vi "LJStreamM read and log.vi"(0 "# Channels":i32=100 min=1, 1 "Scan Rate (Hz)":dbl=500.0 format="%.3f", 2 "# Scans On Graph":i32=1000 min=0, 3 "Update Channel Ref":bool, 4 "LJStreamM Front Panel References":T2, 5 "(LJM) Error In":errorcluster, 6 "Row Modification Options":T1={" Row #"=1, "Delete Row"=FALSE, "Insert Row"=FALSE} {"Row #" min=0 max=95}, 8 "Handle In":i32=43, 10 "start stream":bool caption="Start Stream") -> (9 "Handle Out":i32=43, 14 "Raw Value":dbl[](array[numeric])=[-0.0013667265884578228, 0.9637618064880371, -0.6710270047187805, -1.0797535181045532, -2.244410514831543, -2.9202396869659424, -3.8373279571533203, -4.381304740905762, -5.186929702758789, -5.547481536865234, -6.286360263824463, -6.849207401275635, -8.288508415222168, -9.301578521728516, 1.8125708103179932, -0.0013901632046326995, -0.0013901632046326995, -0.0014061988331377506, -0.001392630278132856, -0.0014173004310578108, -0.0013457569293677807, -0.0013704270822927356, -0.0013149193255230784, -0.0013260208070278168, -1.6386336088180542, -1.2051987648010254, -0.7538595199584961, -0.2919749915599823, 0.20884576439857483, 0.6676713228225708, 1.1433043479919434, 1.6328012943267822, -0.7485023736953735, -0.28742581605911255, 0.18301406502723694, 0.6747994422912598, 1.1796000003814697, 1.6914348602294922, 2.204704523086548, 2.7171919345855713, 0.29239073395729065, 0.7711177468299866, 1.2827318906784058, 1.7454545497894287, 2.2245850563049316, 2.724728584289551, 3.220463991165161, 3.7060885429382324, 1.3471759557724, 1.8994848728179932, 2.4582371711730957, 3.017115592956543, 3.568817377090454, 4.132509231567383, 4.696534633636475, 5.25940465927124, 2.4371588230133057, 2.9621644020080566, 3.493621826171875, 4.033999919891357, 4.572134494781494, 5.092087745666504, 5.614201545715332, 6.141404151916504, 3.54797101020813, 4.116397857666016, 4.69553279876709, 5.2544169425964355, 5.819548606872559, 6.3801727294921875, 6.980928897857666, 7.524782180786133, 4.545636177062988, 5.073090553283691, 5.603622913360596, 6.125936508178711, 6.640289306640625, 7.1512274742126465, 7.6685028076171875, 8.177851676940918, 5.359930992126465, 5.915652275085449, 6.470480442047119, 7.029056549072266, 7.650485038757324, 8.190069198608398, 8.722926139831543, 9.247248649597168, 6.308043956756592, 6.83182430267334, 7.344102382659912, 7.853759765625, 8.360687255859375, 8.86483383178711, 9.365800857543945, 9.856183052062988, 6.392543792724609, 6.943355083465576, 7.586986064910889, 8.126357078552246] format="%.6f", 15 "Scaled Value":dbl[](array[numeric])=[-0.0013667265884578228, 0.9637618064880371, -0.6710270047187805, -1.0797535181045532, -2.244410514831543, -2.9202396869659424, -3.8373279571533203, -4.381304740905762, -5.186929702758789, -5.547481536865234, -6.286360263824463, -6.849207401275635, -8.288508415222168, -9.301578521728516, 1.8125708103179932, -0.0013901632046326995, -0.0013901632046326995, -0.0014061988331377506, -0.001392630278132856, -0.0014173004310578108, -0.0013457569293677807, -0.0013704270822927356, -0.0013149193255230784, -0.0013260208070278168, -1.6386336088180542, -1.2051987648010254, -0.7538595199584961, -0.2919749915599823, 0.20884576439857483, 0.6676713228225708, 1.1433043479919434, 1.6328012943267822, -0.7485023736953735, -0.28742581605911255, 0.18301406502723694, 0.6747994422912598, 1.1796000003814697, 1.6914348602294922, 2.204704523086548, 2.7171919345855713, 0.29239073395729065, 0.7711177468299866, 1.2827318906784058, 1.7454545497894287, 2.2245850563049316, 2.724728584289551, 3.220463991165161, 3.7060885429382324, 1.3471759557724, 1.8994848728179932, 2.4582371711730957, 3.017115592956543, 3.568817377090454, 4.132509231567383, 4.696534633636475, 5.25940465927124, 2.4371588230133057, 2.9621644020080566, 3.493621826171875, 4.033999919891357, 4.572134494781494, 5.092087745666504, 5.614201545715332, 6.141404151916504, 3.54797101020813, 4.116397857666016, 4.69553279876709, 5.2544169425964355, 5.819548606872559, 6.3801727294921875, 6.980928897857666, 7.524782180786133, 4.545636177062988, 5.073090553283691, 5.603622913360596, 6.125936508178711, 6.640289306640625, 7.1512274742126465, 7.6685028076171875, 8.177851676940918, 5.359930992126465, 5.915652275085449, 6.470480442047119, 7.029056549072266, 7.650485038757324, 8.190069198608398, 8.722926139831543, 9.247248649597168, 6.308043956756592, 6.83182430267334, 7.344102382659912, 7.853759765625, 8.360687255859375, 8.86483383178711, 9.365800857543945, 9.856183052062988, 6.392543792724609, 6.943355083465576, 7.586986064910889, 8.126357078552246] format="%.6f", 16 "Last Error Message":string="No Error", 17 "Last Error Message Status":bool, 18 "Channel Setup Reference Out":refnum<vi>, 19 "(LJM) Error Out":errorcluster)   [LabVIEW 2026]
uses:
  Common Logger Controls/Channel Setup.ctl
  LJStreamM Front Panel References.ctl
  Common Logger Controls/Row Modification Options.ctl
  Common Logger VIs/LJM logger Globals.vi
panel:
  in  "Channel Setup":T3={"Name"=["AIN0", "AIN1", "AIN2", "AIN3", "AIN4", "AIN5", "AIN6", "AIN7", "AIN8", "AIN9", "AIN10", "AIN11", "AIN12", "AIN13", "AIN14", "AIN15", "AIN16", "AIN17", "AIN18", "AIN19", "AIN20", "AIN21", "AIN22", "AIN23", "AIN24", "AIN25", "AIN26", "AIN27", "AIN28", "AIN29", "AIN30", "AIN31", "AIN32", "AIN33", "AIN34", "AIN35", "AIN36", "AIN37", "AIN38", "AIN39", "AIN40", "AIN41", "AIN42", "AIN43", "AIN44", "AIN45", "AIN46", "AIN47", "AIN48", "AIN49", "AIN50", "AIN51", "AIN52", "AIN53", "AIN54", "AIN55", "AIN56", "AIN57", "AIN58", "AIN59", "AIN60", "AIN61", "AIN62", "AIN63", "AIN64", "AIN65", "AIN66", "AIN67", "AIN68", "AIN69", "AIN70", "AIN71", "AIN72", "AIN73", "AIN74", "AIN75", "AIN76", "AIN77", "AIN78", "AIN79", "AIN80", "AIN81", "AIN82", "AIN83", "AIN84", "AIN85", "AIN86", "AIN87", "AIN88", "AIN89", "AIN90", "AIN91", "AIN92", "AIN93", "AIN94", "AIN95", "AIN96", "AIN97", "AIN98", "AIN99"], "", "Scaling Equation"=["y=a", "y=b", "y=c", "y=d", "y=e", "y=f", "y=g", "y=h", "y=i", "y=j", "y=k", "y=l", "y=m", "y=n", "y=o", "y=p", "y=q", "y=r", "y=s", "y=t", "y=u", "y=v", "y=w", "y=x", "y=y", "y=z", "y=a2", "y=b2", "y=c2", "y=d2", "y=e2", "y=f2", "y=g2", "y=h2", "y=i2", "y=j2", "y=k2", "y=l2", "y=m2", "y=n2", "y=o2", "y=p2", "y=q2", "y=r2", "y=s2", "y=t2", "y=u2", "y=v2", "y=w2", "y=x2", "y=y2", "y=z2", "y=a3", "y=b3", "y=c3", "y=d3", "y=e3", "y=f3", "y=g3", "y=h3", "y=i3", "y=j3", "y=k3", "y=l3", "y=m3", "y=n3", "y=o3", "y=p3", "y=q3", "y=r3", "y=s3", "y=t3", "y=u3", "y=v3", "y=w3", "y=x3", "y=y3", "y=z3", "y=a4", "y=b4", "y=c4", "y=d4", "y=e4", "y=f4", "y=g4", "y=h4", "y=i4", "y=j4", "y=k4", "y=l4", "y=m4", "y=n4", "y=o4", "y=p4", "y=q4", "y=r4", "y=s4", "y=t4", "y=u4", "y=v4"], "", "Graph?"=[TRUE, TRUE, TRUE, TRUE, FALSE, FALSE, FALSE, FALSE, FALSE, FALSE, FALSE, FALSE, FALSE, FALSE, FALSE, FALSE, FALSE, FALSE, FALSE, FALSE, FALSE, FALSE, FALSE, FALSE, FALSE, FALSE, FALSE, FALSE, FALSE, FALSE, FALSE, FALSE, FALSE, FALSE, FALSE, FALSE, FALSE, FALSE, FALSE, FALSE, FALSE, FALSE, FALSE, FALSE, FALSE, FALSE, FALSE, FALSE, FALSE, FALSE, FALSE, FALSE, FALSE, FALSE, FALSE, FALSE, FALSE, FALSE, FALSE, FALSE, FALSE, FALSE, FALSE, FALSE, FALSE, FALSE, FALSE, FALSE, FALSE, FALSE, FALSE, FALSE, FALSE, FALSE, FALSE, FALSE, FALSE, FALSE, FALSE, FALSE, FALSE, FALSE, FALSE, FALSE, FALSE, FALSE, FALSE, FALSE, FALSE, FALSE, FALSE, FALSE, FALSE, FALSE, FALSE, FALSE, FALSE, FALSE, FALSE, FALSE]}
  # "0"
  # "1"
  # "2"
  # "3"
  # "4"
  # "5"
  # "6"
  # "7"
  # "8"
  # "9"
  # "10"
  # "11"
  # "12"
  # "13"
  # "14"
  # "15"
  # "16"
  # "17"
  # "18"
  # "19"
  # "20"
  # "21"
  # "22"
  # "23"
  # "24"
  # "25"
  # "26"
  # "27"
  # "28"
  # "29"
  # "30"
  # "31"
  # "32"
  # "33"
  # "34"
  # "35"
  # "36"
  # "37"
  # "38"
  # "39"
  # "40"
  # "41"
  # "42"
  # "43"
  # "44"
  # "45"
  # "46"
  # "47"
  # "48"
  # "49"
  # "50"
  # "51"
  # "52"
  # "53"
  # "54"
  # "55"
  # "56"
  # "57"
  # "58"
  # "59"
  # "60"
  # "61"
  # "62"
  # "63"
  # "64"
  # "65"
  # "66"
  # "67"
  # "68"
  # "69"
  # "70"
  # "71"
  # "72"
  # "73"
  # "74"
  # "75"
  # "76"
  # "77"
  # "78"
  # "79"
  # "80"
  # "81"
  # "82"
  # "83"
  # "84"
  # "85"
  # "86"
  # "87"
  # "88"
  # "89"
  # "90"
  # "91"
  # "92"
  # "93"
  # "94"
  # "95"
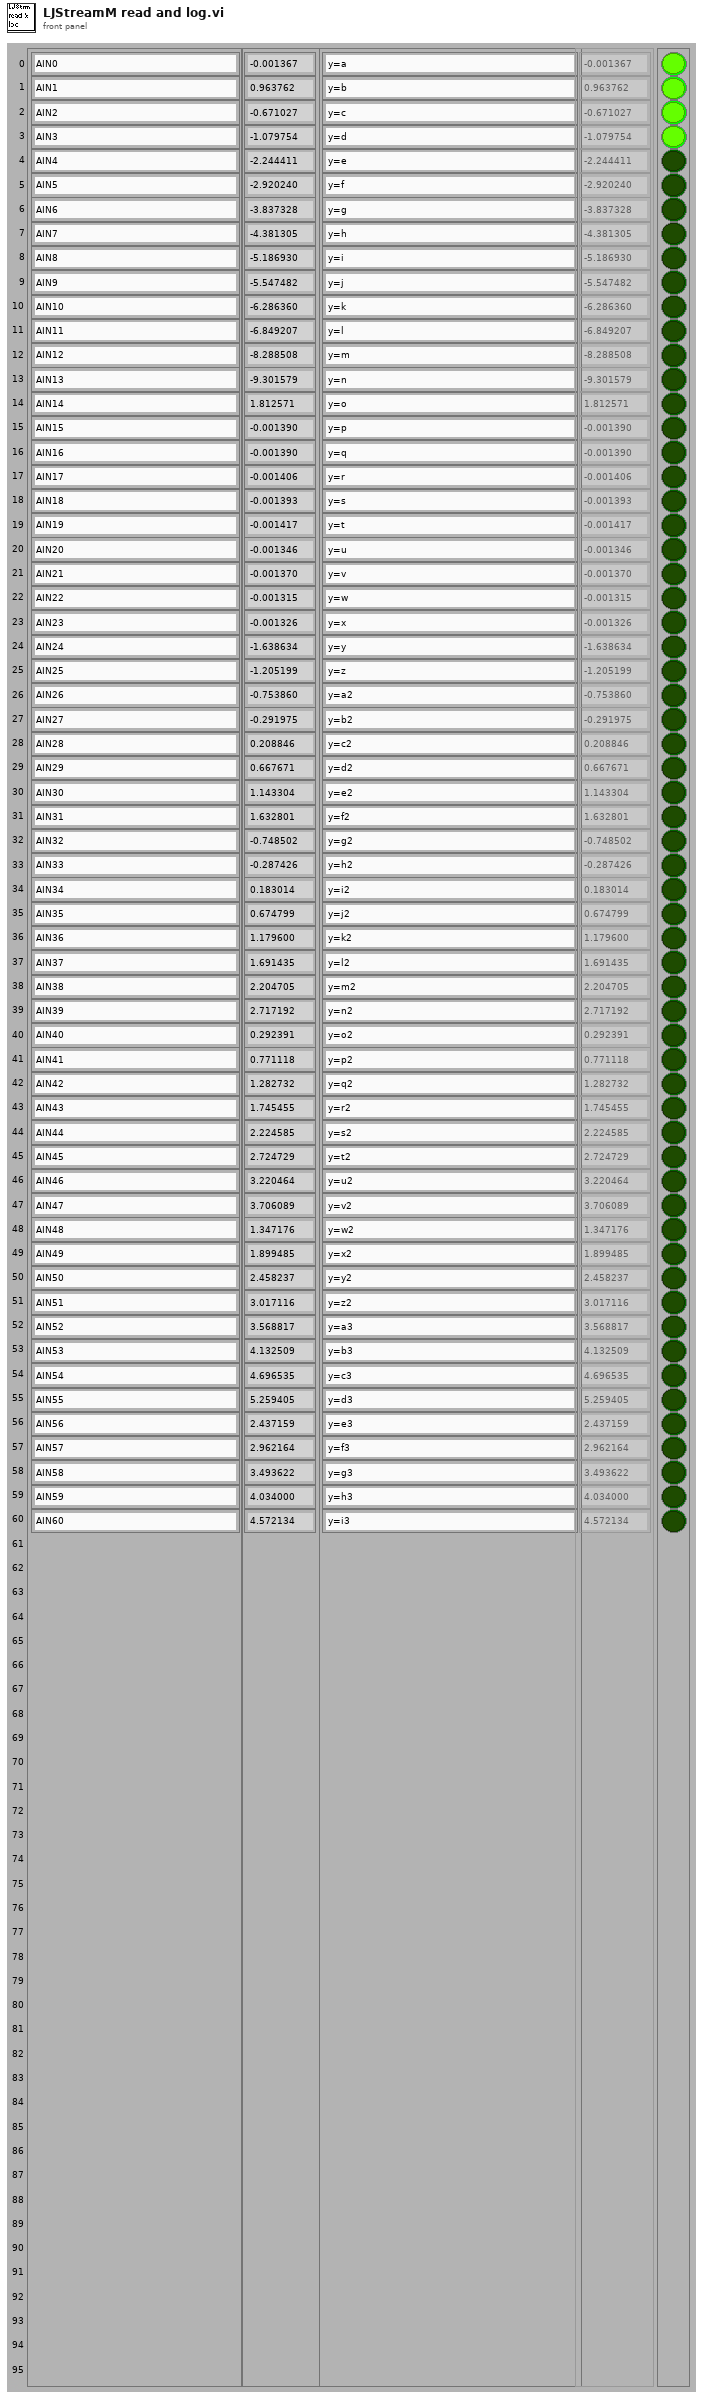
[diagram p1: front panel]
types:
  T1 = typedef "Row Modification Options.ctl" = cluster{" Row #":i32, "Delete Row":bool, "Insert Row":bool}
  T2 = typedef "LJStreamM Front Panel References.ctl" = cluster{"# Scans Read":refnum<vi>, "# of iterations Ref":refnum<vi>, "ms Per Loop Ref":refnum<vi>, "DeviceScanBacklog Ref":refnum<vi>, "LJMScanBacklog Ref":refnum<vi>, "Stop Stream Ref":refnum<vi>, "Disable Scaling* Ref":refnum<vi>, "Write To File Ref":refnum<vi>, "Current Data File Ref":refnum<vi>, "Waveform Graph Ref":refnum<vi>, "Data File Prefix Ref":refnum<vi>, "Max File Size (Bytes) Ref":refnum<vi>, "Channel Setup Reference In":refnum<vi>}
  T3 = typedef "Channel Setup.ctl" = cluster{"Name":string[], string, "Scaling Equation":string[], string, "Graph?":bool[]}
  T4 = cluster{"Name":string[], string, "Scaling Equation":string[], string, "Graph?":bool[]}
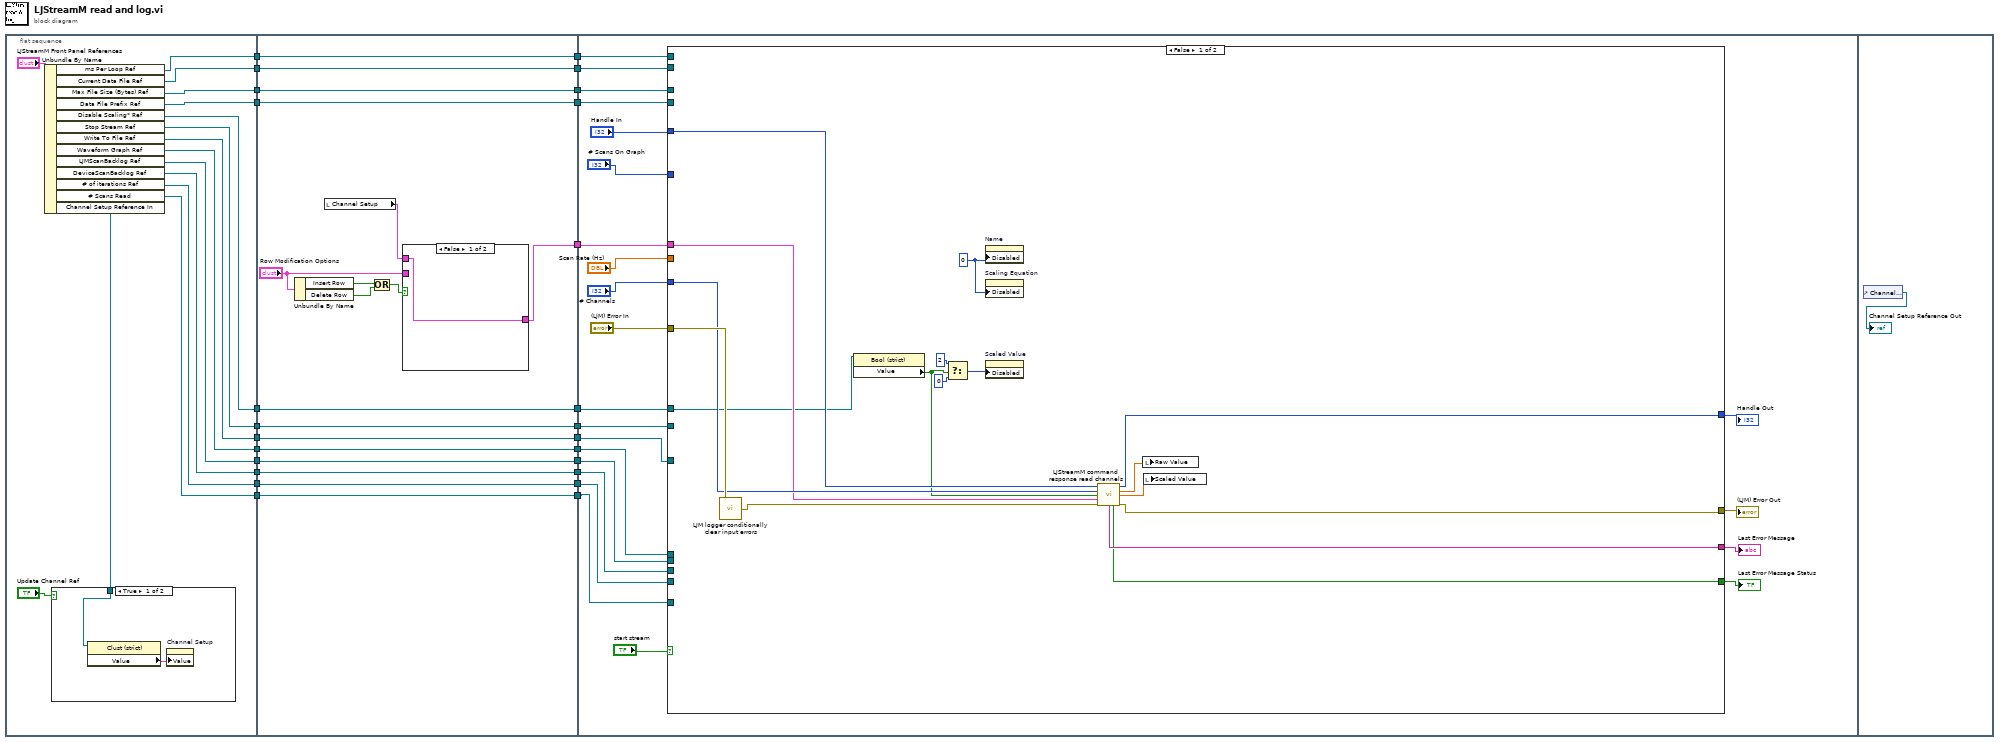
[diagram p0: block diagram]
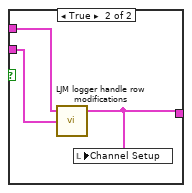
[diagram p3: hidden frame]
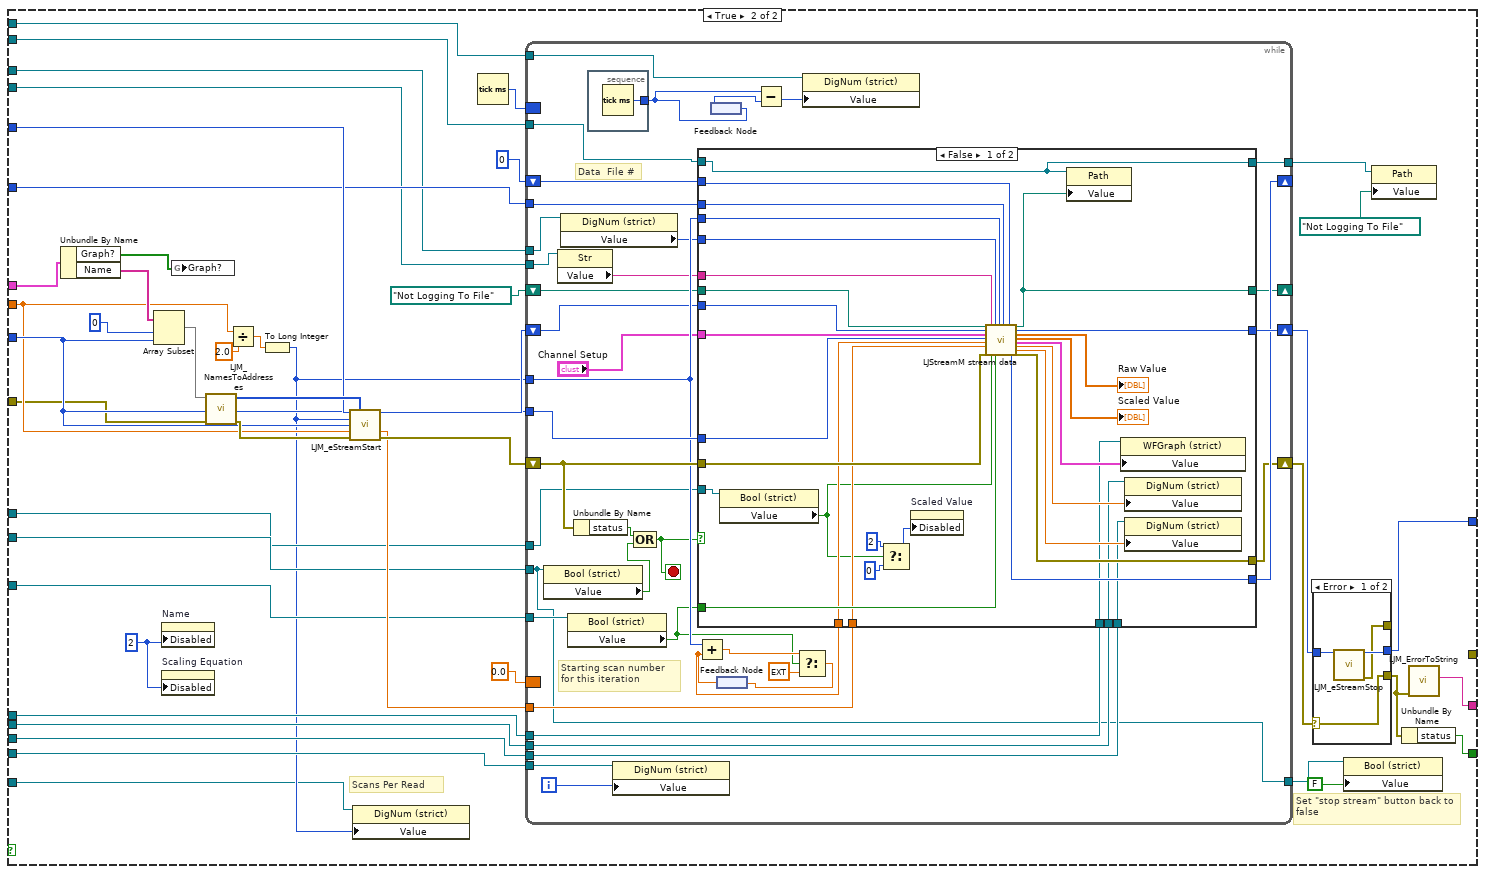
[diagram p4: hidden frame]
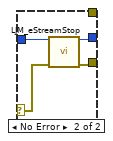
[diagram p6: hidden frame]
diagram:
  n1 = flat-sequence {
    tunnel: [w38] -> w25
    tunnel: [w37] -> w23
    tunnel: [w36] -> w21
    tunnel: [w35] -> w19
    tunnel: [w34] -> w17
    tunnel: [w33] -> w15
    tunnel: [w32] -> w13
    tunnel: [w31] -> w11
    tunnel: [w29] -> w9
    tunnel: [w30] -> w7
    tunnel: [w28] -> w5
    tunnel: [w27] -> w3
    tunnel: w25 -> [w60]
    tunnel: [w60] -> w24
    tunnel: w23 -> [w59]
    tunnel: [w59] -> w22
    tunnel: w21 -> [w58]
    tunnel: [w58] -> w20
    tunnel: w19 -> [w57]
    tunnel: [w57] -> w18
    tunnel: w17 -> [w56]
    tunnel: [w56] -> w16
    tunnel: w15 -> [w55]
    tunnel: [w55] -> w14
    tunnel: w13 -> [w54]
    tunnel: [w54] -> w12
    tunnel: w11 -> [w53]
    tunnel: [w53] -> w10
    tunnel: w9 -> [w52]
    tunnel: [w52] -> w8
    tunnel: w7 -> [w51]
    tunnel: [w51] -> w6
    tunnel: w5 -> [w50]
    tunnel: [w50] -> w4
    tunnel: w3 -> [w49]
    tunnel: [w49] -> w2
    tunnel: [w44] -> w1
    tunnel: w24 -> [w77]
    tunnel: w22 -> [w76]
    tunnel: w20 -> [w75]
    tunnel: w18 -> [w74]
    tunnel: w16 -> [w73]
    tunnel: w14 -> [w72]
    tunnel: w12 -> [w71]
    tunnel: w10 -> [w70]
    tunnel: w8 -> [w69]
    tunnel: w6 -> [w68]
    tunnel: w4 -> [w67]
    tunnel: w2 -> [w66]
    tunnel: w1 -> [w65]
    frame #0 {
      n2 = Unbundle By Name("LJStreamM Front Panel References") -> ("ms Per Loop Ref"=w38:refnum<vi>, "Current Data File Ref"=w37:refnum<vi>, "Max File Size (Bytes) Ref"=w28:refnum<vi>, "Data File Prefix Ref"=w27:refnum<vi>, "Disable Scaling* Ref"=w29:refnum<vi>, "Stop Stream Ref"=w31:refnum<vi>, "Write To File Ref"=w32:refnum<vi>, "Waveform Graph Ref"=w33:refnum<vi>, "LJMScanBacklog Ref"=w34:refnum<vi>, "DeviceScanBacklog Ref"=w35:refnum<vi>, "# of iterations Ref"=w36:refnum<vi>, "# Scans Read"=w30:refnum<vi>, "Channel Setup Reference In"=w26:refnum<vi>)
      n3 = case shown="True" "Update Channel Ref" {
        tunnel: w26 -> [w41 _]
        frame True {
          n4 = property class="Clust (strict)"(reference=w41) -> ("Value"=w42:T4)  [unwired: 1 in, 2 out]
          n5 = property on="Channel Setup" class="Clust (strict)"("Value"=w42) -> ()  [unwired: 2 in, 2 out]
        }
        frame False {
        }
      }
    }
    frame #1 {
      n6 = Unbundle By Name("Row Modification Options") -> ("Insert Row"=w45:bool, "Delete Row"=w46:bool)
      n7 = local read "Channel Setup"() -> (w43:T3)
      n8 = Or(x=w45, y=w46) -> (x .or. y?=w47:bool)
      n9 = case shown="False" w47 {
        tunnel: "Row Modification Options" -> [_ w64]
        tunnel: [w61 w63] -> w44
        tunnel: w43 -> [w61 w62]
        frame False {
        }
        frame True {
          n10 = call "LJM logger handle row modifications.vi"("Row Modification Options"=w64, "Channel Setup"=w62) -> ("Channel Setup Out"=w63:T3)  [unwired: 3 in]
          n11 = local write "Channel Setup"(w63) -> ()
        }
      }
    }
    frame #2 {
      n12 = case shown="False" "start stream" {
        tunnel: [w103 _] -> w80
        tunnel: [w102 w149] -> w81
        tunnel: "Handle In" -> [w100 w142]
        tunnel: "(LJM) Error In" -> [w104 w127]
        tunnel: w65 -> [w98 w132]
        tunnel: "# Scans On Graph" -> [_ w130]
        tunnel: "# Channels" -> [w101 w129]
        tunnel: "Scan Rate (Hz)" -> [_ w128]
        tunnel: [w96 w125] -> w79
        tunnel: [w97 w124] -> w78
        tunnel: w77 -> [_ w123]
        tunnel: w76 -> [_ w122]
        tunnel: w75 -> [_ w121]
        tunnel: w74 -> [_ w120]
        tunnel: w73 -> [_ w119]
        tunnel: w72 -> [_ w118]
        tunnel: w71 -> [_ w117]
        tunnel: w70 -> [_ w116]
        tunnel: w69 -> [w93 w115]
        tunnel: w68 -> [_ w111]
        tunnel: w67 -> [_ w107]
        tunnel: w66 -> [_ w106]
        frame False {
          w88 = u8 0 ("Disabled")
          n13 = call "LJM logger conditionally clear input errors.vi"("error in"=w104) -> ("error out"=w99:errorcluster)
          n14 = property on="Property Node" class="Bool (strict)"(reference=w93) -> ("Value"=w89:bool)  [unwired: 1 in, 2 out]
          n15 = Select(t=u8 2, s=w89, f=u8 0) -> (s? t:f=w90:u8)
          n16 = property on="Name" class="Arr (strict)"("Disabled"=w88) -> ()  [unwired: 2 in, 2 out]
          n17 = property on="Scaling Equation" class="Arr (strict)"("Disabled"=w88) -> ()  [unwired: 2 in, 2 out]
          n18 = property on="Scaled Value" class="Arr (strict)"("Disabled"=w90) -> ()  [unwired: 2 in, 2 out]
          n19 = call "LJStreamM command response read channels.vi"("Handle In"=w100, "# Channels"=w101, "Disable Scaling"=w89, "Channel Setup In"=w98, "Error In"=w99) -> ("Handle Out"=w102:i32, "Raw Data"=w94:dbl[], "Scaled Data"=w95:dbl[], "Error Message"=w97:string, "Error Message Status"=w96:bool, "(LJM) Error Out"=w103:errorcluster)  [unwired: 5 in]
          n20 = local write "Raw Value"(w94) -> ()
          n21 = local write "Scaled Value"(w95) -> ()
        }
        frame True {
          w105 = u8 2 ("Disabled")
          # "Scans Per Read"
          # "Set \"stop stream\" button back to false"
          n22 = Unbundle By Name(w132) -> ("Graph?"=w110:bool[], "Name"=w131:string[])
          n23 = Array Subset(array=w131, index=0 ("Array Index"), length=w129) -> (w146:string[])
          n24 = property on="Name" class="Arr (strict)"("Disabled"=w105) -> ()  [unwired: 2 in, 2 out]
          n25 = property on="Scaling Equation" class="Arr (strict)"("Disabled"=w105) -> ()  [unwired: 2 in, 2 out]
          n26 = global write "LJM logger Globals.vi" "Graph?"(w110) -> ()
          n27 = call "LJM_NamesToAddresses.vi"("NumFrames (Auto-Detect)"=w129, "error in"=w127, "aNames"=w146) -> ("error out"=w147:errorcluster, "aAddresses"=w145:i32[])  [unwired: 6 in, 1 out]
          n28 = Divide(x=w128, y=2.0) -> (x/y=w143:dbl)
          n29 = To Long Integer(number=w143) -> (32bit integer=w112:i32)
          n30 = call "LJM_eStreamStart.vi"("Handle In"=w142, "aScanList"=w145, "ScansPerRead"=w112, "NumAddresses (Auto-Detect)"=w129, "ScanRate"=w128, "error in"=w147) -> ("Handle Out"=w134:i32, "Actual ScanRate"=w137:dbl, "error out"=w141:errorcluster)  [unwired: 4 in, 3 out]
          n31 = property class="DigNum (strict)"(reference=w111, "Value"=w112) -> ()  [unwired: 1 in, 2 out]
          n32 = Tick Count (ms)() -> (millisecond timer value=w139:u32)
          n33 = while {
            tunnel: w129 -> [w188]
            tunnel: w137 -> [w187]
            tunnel: w112 -> [w179]
            shift-right: [w175] -> _
            shift-left: 0 ("# Scans Read") -> [w176]
            tunnel: w130 -> [w173]
            shift-right: [w186] -> w140
            shift-left: w134 -> [w171]
            shift-right: [w155] -> w133
            shift-left: w141 -> [w183]
            shift-right: [w170] -> _
            shift-left: path "Not Logging To File" ("Current Data File Out") -> [w172]
            tunnel: w123 -> [w169]
            tunnel: w122 -> [w167]
            tunnel: w121 -> [w166]
            tunnel: w120 -> [w160]
            tunnel: w119 -> [w161]
            tunnel: w118 -> [w162]
            tunnel: w117 -> [w159]
            tunnel: w116 -> [w158]
            tunnel: w115 -> [w163]
            tunnel: [w158] -> w113
            tunnel: [w154] -> w108
            tunnel: w107 -> [w151]
            tunnel: w106 -> [w152]
            border: w139 -> [_]
            border: 0.0 ("y") -> [_]
            i -> [w156]
            stop <- w174 stop-if-true
            # "Starting scan number for this iteration"
            # "Data  File #"
            n34 = property class="Bool (strict)"(reference=w158) -> ("Value"=w164:bool)  [unwired: 1 in, 2 out]
            n35 = property class="Str"(reference=w152) -> ("Value"=w153:string)  [unwired: 1 in, 2 out]
            n36 = property class="DigNum (strict)"(reference=w151) -> ("Value"=w150:i32)  [unwired: 1 in, 2 out]
            n37 = property class="Bool (strict)"(reference=w159) -> ("Value"=w165:bool)  [unwired: 1 in, 2 out]
            n38 = Unbundle By Name(w183) -> ("status"=w182:bool)
            n39 = stacked-sequence {
              tunnel: [w225] -> w184
              frame #0 {
                n40 = Tick Count (ms)() -> (millisecond timer value=w225:u32)
              }
            }
            n41 = property class="DigNum (strict)"(reference=w166, "Value"=w156) -> ()  [unwired: 1 in, 2 out]
            n42 = Compound Arithmetic op=OR(w182, w164) -> (w174:bool)
            n43 = feedback-in #1(w184) -> ()
            n44 = feedback #1() -> (w185:u32)
            n45 = feedback #2() -> (w177:ext)
            n46 = Add(x=w179, y=w177) -> (x+y=w180:ext)
            n47 = case shown="False" w174 {
              tunnel: "Channel Setup" -> [w219 _]
              tunnel: w188 -> [w218 _]
              tunnel: w187 -> [w211 _]
              tunnel: w179 -> [w213 _]
              tunnel: [w217 w223] -> w155
              tunnel: [w216 w224] -> w186
              tunnel: w171 -> [w215 w224]
              tunnel: w183 -> [w214 w223]
              tunnel: w165 -> [w212 _]
              tunnel: w177 -> [w210 _]
              tunnel: w176 -> [w209 w222]
              tunnel: [w208 w222] -> w175
              tunnel: w173 -> [w207 _]
              tunnel: w172 -> [w206 w221]
              tunnel: [w204 w221] -> w170
              tunnel: w153 -> [w205 _]
              tunnel: w167 -> [w190 w220]
              tunnel: w163 -> [w203 _]
              tunnel: w162 -> [w199 _]
              tunnel: w161 -> [w198 _]
              tunnel: w160 -> [w197 _]
              tunnel: [w190 w220] -> w154
              tunnel: w150 -> [w189 _]
              frame False {
                n48 = property class="Bool (strict)"(reference=w203) -> ("Value"=w191:bool)  [unwired: 1 in, 2 out]
                n49 = Select(t=u8 2, s=w191, f=u8 0) -> (s? t:f=w194:u8)
                n50 = property on="Scaled Value" class="Arr (strict)"("Disabled"=w194) -> ()  [unwired: 2 in, 2 out]
                n51 = call "LJStreamM stream data.vi"("Data File Reference In"=w206, "Handle In"=w215, "Channel Setup"=w219, "# Channels"=w218, "Starting Scan Number"=w210, "Scan Rate"=w211, "Error In"=w214, "Data File Prefix"=w205, "Disable Scaling*"=w191, "Max File Size (Bytes)"=w189, "Write To File"=w212, "Scans Per Read"=w213, "# Scans On Graph"=w207, "Starting #"=w209) -> ("Data File #"=w208:u32, "Data File Reference Out"=w204:path, "Handle Out"=w216:i32, "Raw Value"=→"Raw Value":dbl[], "Scaled Value"=→"Scaled Value":dbl[], "Waveform Graph"=w200:cluster{dbl, dbl, dbl[][]}, "LJMScanBacklog"=w201:dbl, "DeviceScanBacklog"=w202:dbl, "Error Out"=w217:errorcluster)  [unwired: 5 in]
                n52 = property class="Path"(reference=w190, "Value"=w204) -> ()  [unwired: 1 in, 2 out]
                n53 = property class="WFGraph (strict)"(reference=w199, "Value"=w200) -> ()  [unwired: 1 in, 2 out]
                n54 = property class="DigNum (strict)"(reference=w198, "Value"=w201) -> ()  [unwired: 1 in, 2 out]
                n55 = property class="DigNum (strict)"(reference=w197, "Value"=w202) -> ()  [unwired: 1 in, 2 out]
              }
              frame True {
              }
            }
            n56 = Subtract(x=w184, y=w185) -> (x-y=w168:u32)
            n57 = Select(t=w180, s=w165, f=ext 0.0) -> (s? t:f=w178:ext)
            n58 = feedback-in #2(w178) -> ()
            n59 = property class="DigNum (strict)"(reference=w169, "Value"=w168) -> ()  [unwired: 1 in, 2 out]
          }
          n60 = case shown="Error" w133 {
            selector: w133 -> [w227 w230]
            tunnel: w140 -> [w229 w233]
            tunnel: [w227 w232] -> w126
            tunnel: [w228 w231] -> w149
            tunnel: [w226 _] -> _
            frame Error {
              n61 = call "LJM_eStreamStop.vi"("Handle In"=w229) -> ("Handle Out"=w228:i32, "error out"=w226:errorcluster)  [unwired: 13 in]
            }
            frame No Error {
              n62 = call "LJM_eStreamStop.vi"("Handle In"=w233, "error in"=w230) -> ("Handle Out"=w231:i32, "error out"=w232:errorcluster)  [unwired: 12 in]
            }
          }
          n63 = property class="Bool (strict)"(reference=w113, "Value"=FALSE) -> ()  [unwired: 1 in, 2 out]
          n64 = property class="Path"(reference=w108, "Value"=path "Not Logging To File" ("Current Data File Out")) -> ()  [unwired: 1 in, 2 out]
          n65 = Unbundle By Name(w126) -> ("status"=w125:bool)
          n66 = call "LJM_ErrorToString.vi"("error in"=w126) -> ("String"=w124:string)  [unwired: 10 in]
        }
      }
      "Handle Out" <- w81
      "(LJM) Error Out" <- w80
      "Last Error Message" <- w78
      "Last Error Message Status" <- w79
    }
    frame #3 {
      n67 = control-ref of="Channel Setup"() -> (→"Channel Setup Reference Out":refnum<vi>)
    }
  }
